vi "cold storage.vi"() -> (2 "Subject 2":string="1-Abad Fisheries Private Limited \\n12")   [LabVIEW 2013]
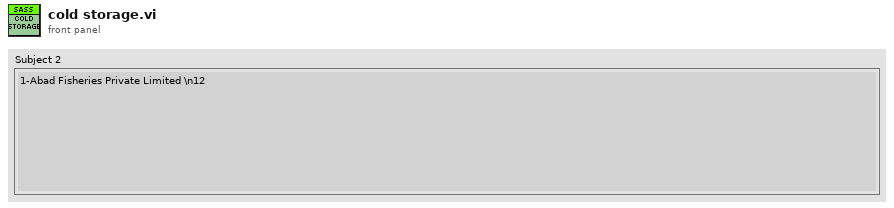
[diagram p1: front panel]
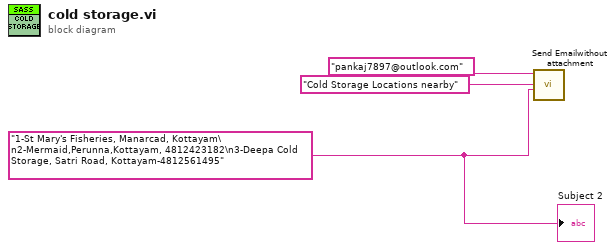
[diagram p0: block diagram]
diagram:
  w1 = "1-St Mary's Fisheries, Manarcad, Kottayam\n2-Mermaid,Perunna,Kottayam, 4812423182\n3-Deepa Cold Storage, Satri Road, Kottayam-4812561495" ("Subject 2")
  n1 = call "Send Emailwithout attachment.vi"("To: 2"="pankaj7897@outlook.com", "Subject 2"="Cold Storage Locations nearby", "Message 2"=w1) -> ()  [unwired: 8 in]
  "Subject 2" <- w1
